vi "ConvertRunOneTestScriptToSSMFormat.vi"(11 "Script in":string[](array[string])) -> (3 "Script out":string[](array[string]))   [LabVIEW 2018]
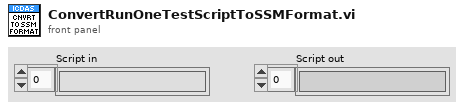
[diagram p1: front panel]
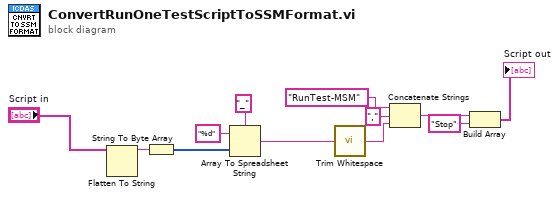
[diagram p0: block diagram]
diagram:
  n1 = Flatten To String(anything="Script in") -> (data string=w6:string)  [unwired: 3 in, 2 out]
  n2 = String To Byte Array(string=w6) -> (unsigned byte array=w7:u8[])
  n3 = Array To Spreadsheet String(delimiter (Tab)="_" ("format string"), array=w7, 3:"%d" ("format string")) -> (spreadsheet string=w10:string)
  n4 = call <vilib>:"Trim Whitespace.vi"("string"=w10) -> ("trimmed string"=w12:string)  [unwired: 1 in]
  n5 = Concatenate Strings("RunTest-MSM" ("Severity"), "," ("string"), w12) -> (w3:string)
  n6 = Build Array(w3, "Stop" ("element")) -> (→"Script out":string[])
